vi "Determine Sector Edge Location.vi"() -> (2 "Left Sector Edge":u8, 3 "Right Sector Edge":u8)   [LabVIEW 2013]
doc: "Takes the average sector intensities and compares each average to the threshold value to determine which sector the edge is located in."
uses:
  Globals/Accumulated Sector Intensity.vi
  Globals/Sector Parameter Global.vi
  <vilib>/rvi/FIFO/Fifo_Resource/nirvififoEmulationReadFpgaImpl.vi
  <vilib>/rvi/DataTransferAndStorage/Container/Common/niFpgaContainerGetUniqueNameForEmu.vi
  <vilib>/rvi/interface/RandomDataEmulation/nirviRandomDataFPGAFIFO.vi
  <vilib>/rvi/interface/RandomDataEmulation/niFpgaRandomDataHandleErrors.vi
  <vilib>/rvi/DataTransferAndStorage/Container/XNode/niFpgaContainer.xnode
  <vilib>/rvi/FIFO/Fifo_Resource/nirvififoEmulationRead.vi
  <vilib>/rvi/interface/RandomDataEmulation/nirviRandomDataFpgaReadWriteTemplate.vi
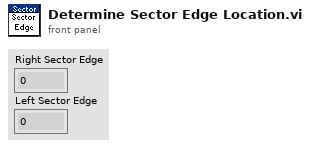
[diagram p1: front panel]
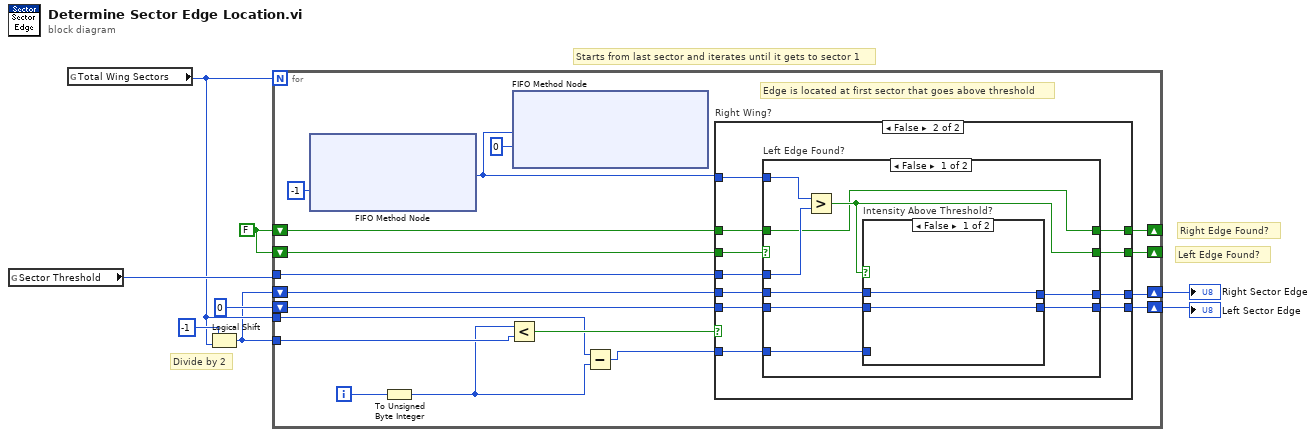
[diagram p0: block diagram]
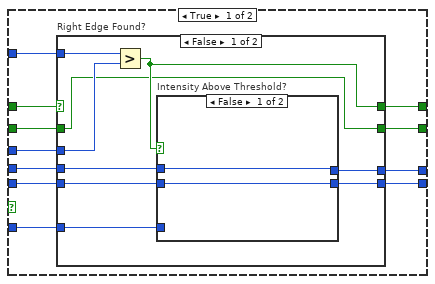
[diagram p2: hidden frame]
diagram:
  w5 = FALSE ("Left Edge Found?")
  # "Starts from last sector and iterates until it gets to sector 1"
  # "Left Edge Found?"
  # "Right Edge Found?"
  # "Divide by 2"
  n1 = global read "Sector Parameter Global.vi" "Sector Threshold"() -> (w3:u8)
  n2 = global read "Accumulated Sector Intensity.vi" "Total Wing Sectors"() -> (w2:u8)
  n3 = Logical Shift(y=i16 -1, x=w2) -> (x << y=w1:u8)
  n4 = for {
    N: w2 -> [_]
    tunnel: w3 -> [w24]
    tunnel: w1 -> [w25]
    shift-right: [w22] -> _
    shift-left: w5 -> [w23]
    shift-right: [w15] -> _
    shift-left: w5 -> [w16]
    shift-right: [w20] -> w8
    shift-left: w1 -> [w19]
    shift-right: [w18] -> w7
    shift-left: u8 0 ("Total Wing Sectors") -> [w17]
    tunnel: w2 -> [w11]
    i -> [w21]
    # "Edge is located at first sector that goes above threshold"
    n5 = xnode ("FIFO Method Node")("Timeout"=-1) -> ("Element"=w14:u8)  [unwired: 1 in, 2 out]
    n6 = To Unsigned Byte Integer(number=w21) -> (unsigned 8bit integer=w10:u8)
    n7 = Less?(x=w10, y=w25) -> (x < y?=w26:bool)
    n8 = xnode ("FIFO Method Node")("Element"=w14, "Timeout"=0) -> ()  [unwired: 1 in, 2 out]
    n9 = Subtract(x=w11, y=w10) -> (x-y=w9:u8)
    n10 = case "Right Wing?" shown="False" w26 {
      tunnel: w14 -> [w36 w65]
      tunnel: w24 -> [w35 w64]
      tunnel: w23 -> [w37 w56]
      tunnel: [w34 w63] -> w22
      tunnel: w9 -> [w33 w62]
      tunnel: [w32 w61] -> w20
      tunnel: w19 -> [w31 w60]
      tunnel: [w30 w59] -> w18
      tunnel: w17 -> [w29 w58]
      tunnel: w16 -> [w28 w57]
      tunnel: [w27 w55] -> w15
      frame True {
        n11 = case "Right Edge Found?" shown="False" w37 {
          selector: w37 -> [_ w51]
          tunnel: w36 -> [w46 _]
          tunnel: w35 -> [w45 _]
          tunnel: [w44 w51] -> w34
          tunnel: w33 -> [w43 _]
          tunnel: [w42 w54] -> w32
          tunnel: w31 -> [w41 w54]
          tunnel: [w40 w53] -> w30
          tunnel: w29 -> [w39 w53]
          tunnel: w28 -> [w38 w52]
          tunnel: [w38 w52] -> w27
          frame False {
            n12 = Greater?(x=w46, y=w45) -> (0:w44:bool)
            n13 = case "Intensity Above Threshold?" shown="False" w44 {
              tunnel: w43 -> [_ w49]
              tunnel: [w48 w49] -> w42
              tunnel: w41 -> [w48 _]
              tunnel: [w47 w50] -> w40
              tunnel: w39 -> [w47 w50]
              frame False {
              }
              frame True {
              }
            }
          }
          frame True {
          }
        }
      }
      frame False {
        n14 = case "Left Edge Found?" shown="False" w57 {
          selector: w57 -> [_ w79]
          tunnel: w65 -> [w74 _]
          tunnel: w64 -> [w73 _]
          tunnel: [w66 w80] -> w63
          tunnel: w62 -> [w72 _]
          tunnel: [w71 w82] -> w61
          tunnel: w60 -> [w70 w82]
          tunnel: [w69 w81] -> w59
          tunnel: w58 -> [w68 w81]
          tunnel: w56 -> [w66 w80]
          tunnel: [w67 w79] -> w55
          frame False {
            n15 = Greater?(x=w74, y=w73) -> (0:w67:bool)
            n16 = case "Intensity Above Threshold?" shown="False" w67 {
              tunnel: w72 -> [_ w77]
              tunnel: [w76 w78] -> w71
              tunnel: w70 -> [w76 w78]
              tunnel: [w75 w77] -> w69
              tunnel: w68 -> [w75 _]
              frame False {
              }
              frame True {
              }
            }
          }
          frame True {
          }
        }
      }
    }
  }
  "Right Sector Edge" <- w8
  "Left Sector Edge" <- w7
